vi "Get 3D Graph Info.vi"(0 "3D Surface":refnum<k7>(container)) -> (1 "Latitude out":dbl format="%.2f", 2 "Longitude out":dbl format="%.2f")   [LabVIEW 2011]
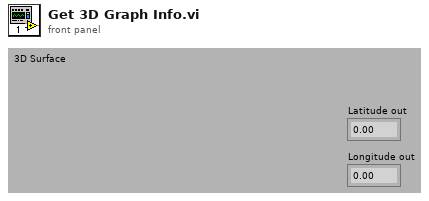
[diagram p1: front panel]
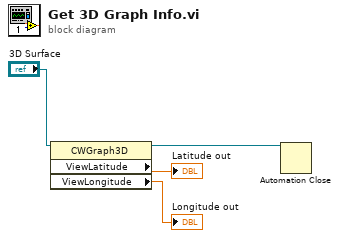
[diagram p0: block diagram]
diagram:
  n1 = property class="CWGraph3D"(reference="3D Surface") -> (reference out=w1:refnum<k7>, "ViewLatitude"=→"Latitude out":dbl, "ViewLongitude"=→"Longitude out":dbl)  [unwired: 1 in, 1 out]
  n2 = Automation Close(5:w1) -> ()  [unwired: 1 in, 1 out]
